vi "testSimpleEventPumping.vi"() -> ()   [LabVIEW 2017]
panel:
  in  "SomeVal":cluster{"TheArray":cluster{"Y":dbl, "X":dbl}[]}
  in  "SimpleNum":dbl
  in  "stop":bool
  out "pID":string
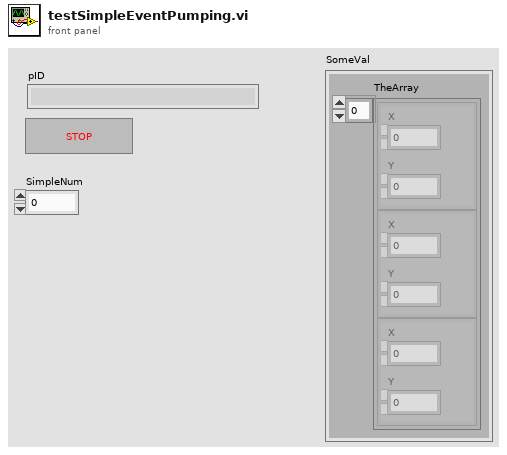
[diagram p1: front panel]
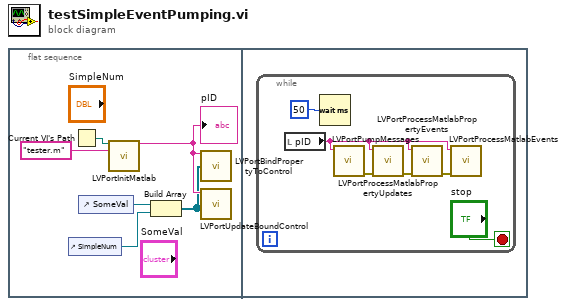
[diagram p0: block diagram]
diagram:
  n1 = flat-sequence {
    frame #0 {
      n2 = control-ref of="SimpleNum"() -> (w2:refnum<vi>)
      n3 = Current VI's Path() -> (path=w6:path)
      n4 = control-ref of="SomeVal"() -> (w3:refnum<vi>)
      n5 = call "LVPortInitMatlab.vi"("Working directory or VI Path"=w6, "Code file name"="tester.m") -> ("ID"=w4:string)  [unwired: 12 in, 1 out]
      "pID" <- w4
      n6 = Build Array(w3, w2) -> (w1:refnum<vi>[])
      n7 = call "LVPortBindPropertyToControl.vi"("pID"=w4, "Controls To Bind"=w1) -> ()  [unwired: 14 in]
      n8 = call "LVPortUpdateBoundControl.vi"("Controls To Update"=w1, "pID"=w4) -> ()  [unwired: 10 in]
    }
    frame #1 {
      n9 = while {
        stop <- "stop" stop-if-true
        n10 = local read "pID"() -> (w9:string)
        n11 = Wait (ms)(milliseconds to wait=u32 50) -> ()  [unwired: 1 out]
        n12 = call "LVPortPumpMessages.vi"("pID"=w9) -> ("error out"=w8:errorcluster)  [unwired: 9 in, 1 out]
        n13 = call "LVPortProcessMatlabPropertyUpdates.vi"("error in"=w8, "pID"=w9) -> ("error out"=w7:errorcluster)  [unwired: 9 in]
        n14 = call "LVPortProcessMatlabPropertyEvents.vi"("error in"=w7, "pID"=w9) -> ("error out"=w10:errorcluster)  [unwired: 9 in]
        n15 = call "LVPortProcessMatlabEvents.vi"("error in"=w10, "pID"=w9) -> ()  [unwired: 9 in, 1 out]
      }
    }
  }
